vi "Add Buffer.vi"(8 "error in":errorcluster, 9 "Name":string, 10 "Buffer":refnum<data-value>, 11 "BufferMap in":refnum<data-value>) -> (0 "error out":errorcluster, 3 "BufferMap":refnum<data-value>)   [LabVIEW 2013, in "CircularBuffer.lvlib" / "VariantBufferMap.lvclass"]
doc: "This VI writes one data element into the current location in the buffer. The location in the buffer is updated automatically."
uses:
  VariantBufferMap.lvclass
  VariantBuffer/VariantBuffer.lvclass
  VariantBufferMap.lvclass/VariantBufferMap.ctl
  VariantBuffer/WriteBufferError.vi
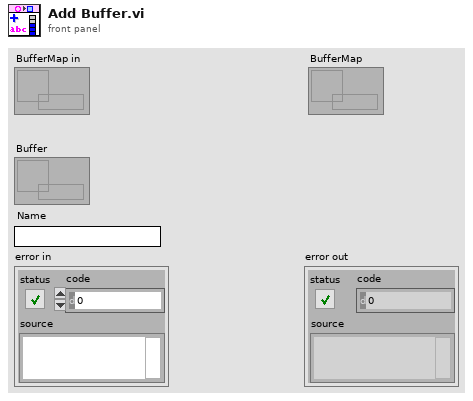
[diagram p1: front panel]
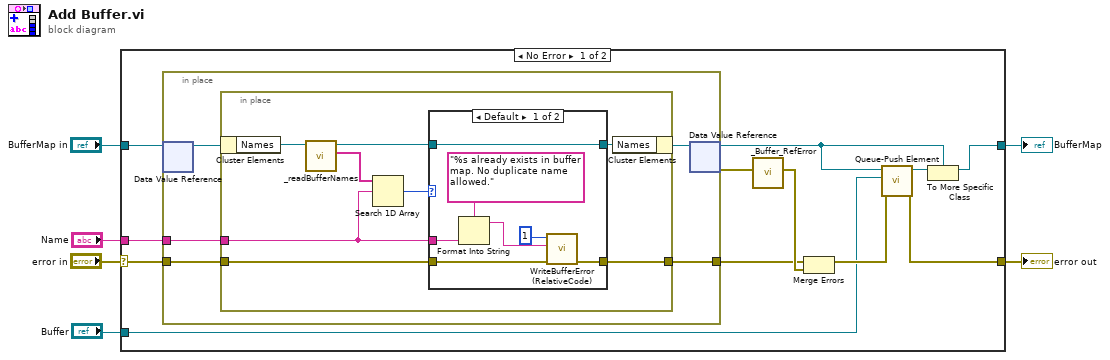
[diagram p0: block diagram]
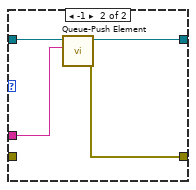
[diagram p2: hidden frame]
diagram:
  n1 = case shown="No Error" "error in" {
    selector: "error in" -> [w9 w44]
    tunnel: "BufferMap in" -> [w15 w43]
    tunnel: [w16 w43] -> w5
    tunnel: [w11 w44] -> w4
    tunnel: "Buffer" -> [w10 _]
    tunnel: "Name" -> [w18 _]
    frame No Error {
      n2 = in-place {
        in-place-border: w18 -> [w21]
        in-place-border: [w20] -> w8
        in-place-border: w9 -> [w19]
        n3 = in-place-dvr #1(w15) -> (w23:refnum<class "VariantBufferMap.lvclass">)  [unwired: 1 out]
        n4 = in-place {
          in-place-border: w21 -> [w29]
          in-place-border: [w28] -> w20
          in-place-border: w19 -> [w24]
          n5 = in-place-cluster #2(w23) -> ("Names"=w31:refnum<data-value>)
          n6 = call "_readBufferNames.vi"("Data Value Reference in"=w31) -> ("Names"=w27:string[], "Data Value Reference out"=w25:refnum<data-value>)  [unwired: 9 in]
          n7 = Search 1D Array(1D array=w27, element=w29) -> (index of element=w26:i32)  [unwired: 1 in]
          n8 = case shown="Default" w26 {
            tunnel: w25 -> [w38 w42]
            tunnel: [w38 w41] -> w30
            tunnel: w29 -> [w34 w40]
            tunnel: [w37 w39] -> w28
            tunnel: w24 -> [w35 _]
            frame Default {
              n9 = Format Into String(format string="%s already exists in buffer map. No duplicate name allowed." ("error message (\"\")"), w34) -> (resulting string=w33:string)  [unwired: 2 in, 1 out]
              n10 = call "WriteBufferError (RelativeCode).vi"("error in (no error)"=w35, "Error message"=w33, "Relative error code (548600 + input)"=1 ("error code (0)")) -> ("error out"=w37:errorcluster)  [unwired: 8 in]
            }
            frame -1 {
              n11 = call "Queue-Push Element.vi"("element"=w40, "Buffer in"=w42) -> ("error out"=w39:errorcluster, "Buffer"=w41:refnum<data-value>)  [unwired: 6 in, 2 out]
            }
          }
          n12 = in-place-cluster #2("Names"=w30) -> (w22:refnum<class "VariantBufferMap.lvclass">)
        }
        n13 = in-place-dvr #1(w22) -> (w7:refnum<data-value>, w14:errorcluster)
      }
      n14 = call "_Buffer_RefError.vi"("error in (no error)"=w14) -> ("error out"=w13:errorcluster)  [unwired: 10 in]
      n15 = Merge Errors(w8, w13) -> (w12:errorcluster)
      n16 = call "Queue-Push Element.vi"("error in"=w12, "element"=w10, "Buffer in"=w7) -> ("error out"=w11:errorcluster, "Buffer"=w17:refnum<data-value>)  [unwired: 5 in, 2 out]
      n17 = To More Specific Class(target class=w7, reference=w17) -> (specific class reference=w16:refnum<data-value>)  [unwired: 1 in, 1 out]
    }
    frame Error {
    }
  }
  "error out" <- w4
  "BufferMap" <- w5
